vi "Database - Setup.vi"(0 "reference in":refnum<class "Database_UUT.lvclass">, 1 "Filepath to Directory of Database":path=path "C:/Users/Test-Eng/Desktop/Temp Test", 2 "Database Name":string="Database", 5 "error in (no error)":errorcluster) -> (14 "reference out":refnum<class "Database_UUT.lvclass">, 15 "Database Filepath":path, 19 "error out":errorcluster)   [LabVIEW 2017, in "Database_UUT.lvclass"]
uses:
  Database_UUT.lvclass
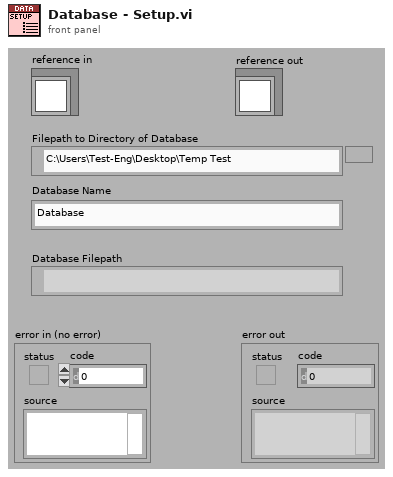
[diagram p1: front panel]
types:
  T1 = enum16{"open", "open or create", "create or replace", "create", "open (read-only)"}
  T2 = typedef "Database.lvclass/ObjectAttributes.ctl" = cluster{"Filepath to Database":path}
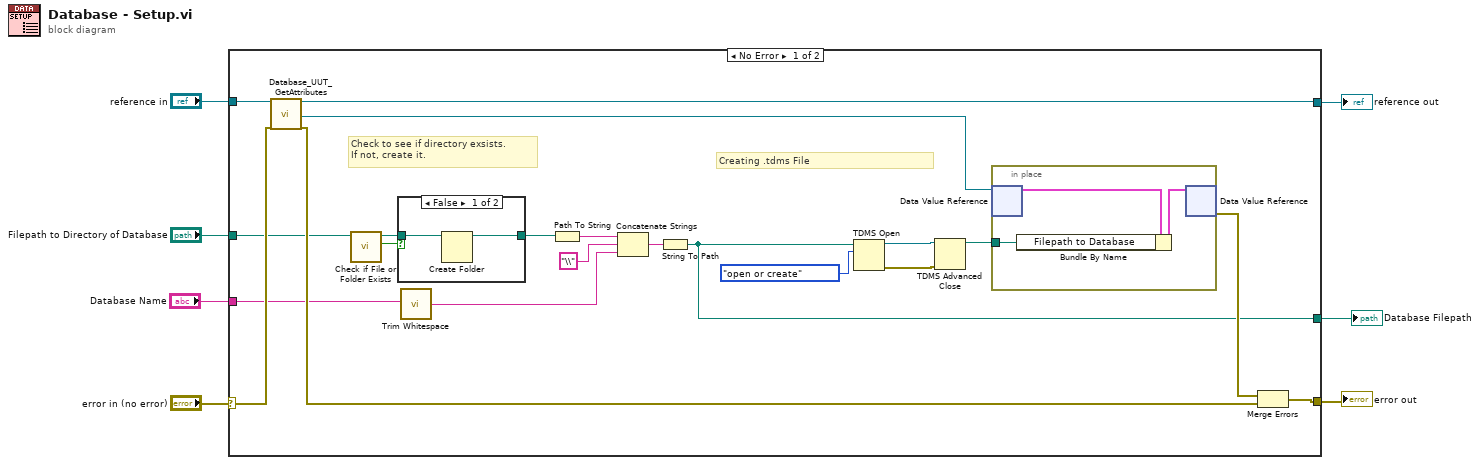
[diagram p0: block diagram]
diagram:
  n1 = case shown="No Error" "error in (no error)" {
    selector: "error in (no error)" -> [w27 w36]
    tunnel: [w24 w36] -> w6
    tunnel: [w25 w35] -> w4
    tunnel: "reference in" -> [w28 w35]
    tunnel: "Filepath to Directory of Database" -> [w19 _]
    tunnel: "Database Name" -> [w9 _]
    tunnel: [w10 _] -> w1
    frame No Error {
      # "Check to see if directory exsists.\nIf not, create it."
      # "Creating .tdms File"
      n2 = call "Database_UUT_GetAttributes.vi"("reference in"=w28, "error in (no error)"=w27) -> ("reference out"=w25:refnum<class "Database_UUT.lvclass">, "DataRef"=w23:refnum<data-value>, "error out"=w22:errorcluster)  [unwired: 14 in, 1 out]
      n3 = call <vilib>:"Check if File or Folder Exists.vi"("path"=w19) -> ("file or folder exists?"=w18:bool, "dup path"=w17:path)  [unwired: 8 in, 1 out]
      n4 = case shown="False" w18 {
        tunnel: w17 -> [w30 w31]
        tunnel: [w29 w31] -> w14
        frame False {
          n5 = Create Folder(path (use dialog)=w30) -> (created path=w29:path)  [unwired: 2 in, 2 out]
        }
        frame True {
        }
      }
      n6 = call <vilib>:"Trim Whitespace.vi"("string"=w9) -> ("trimmed string"=w8:string)  [unwired: 1 in]
      n7 = Path To String(path=w14) -> (string=w13:string)
      n8 = Concatenate Strings(w13, "\\", w8) -> (w11:string)
      n9 = String To Path(string=w11) -> (path=w10:path)
      n10 = TDMS Open(10:T1."open or create" ("operation (0:open)"), 11:w10) -> (0:w21:errorcluster, 3:w20:refnum<k34>)  [unwired: 5 in]
      n11 = TDMS Advanced Close(8:w21, 11:w20) -> (3:w15:path)  [unwired: 2 in, 1 out]
      n12 = in-place {
        in-place-border: w15 -> [w32]
        n13 = in-place-dvr #1(w23) -> (w33:T2)  [unwired: 1 out]
        n14 = Bundle By Name(cluster=w33, "Filepath to Database"=w32) -> (w34:T2)
        n15 = in-place-dvr #1(w34) -> (w26:errorcluster)  [unwired: 1 out]
      }
      n16 = Merge Errors(w26, w22) -> (w24:errorcluster)
    }
    frame Error {
    }
  }
  "error out" <- w6
  "reference out" <- w4
  "Database Filepath" <- w1
